vi "Day 14.vi"() -> ()   [LabVIEW 2025]
panel:
  out "# of sand":i32
  out "cave array":string[][](array[string])
  out "lines array":string[](array[string])
  out "sand pour":i32
  out "Y offset":i32
  out "X":i32
  out "Y":i32
  in  "test":bool
  in  "test input":string="498,4 -> 498,6 -> 496,6\n503,4 -> 502,4 -> 502,9 -> 494,9"
  in  "input":string="487,45 -> 487,38 -> 487,45 -> 489,45 -> 489,42 -> 489,45 -> 491,45 -> 491,39 -> 491,45 -> 493,45 -> 493,39 -> 493,45\n512,90 -> 512,87 -> 512,90 -> 514,90 -> 514,86 -> 514,90 -> 516,90 -> 516,87 -> 516,90 -> 518,90 -> 518,82 -> 518,90 -> 520,90 -> 520,81 -> 520,90 -> 522,90 -> 522,86 -> 522,90 -> 524,90 -> 524,84 -> 524,90 -> 526,90 -> 526,82 -> 526,90 -> 528,90 -> 528,82 -> 528,90\n494,16 -> 499,16\n512,90 -> 512,87 -> 512,90 -> 514,90 -> 514,86 -> 514,90 -> 516,90 -> 516,87 -> 516,90 -> 518,90 -> 518,82 -> 518,90 -> 520,90 -> 520,81 -> 520,90 -> 522,90 -> 522,86 -> 522,90 -> 524,90 -> 524,84 -> 524,90 -> 526,90 -> 526,82 -> 526,90 -> 528,90 -> 528,82 -> 528,90\n505,57 -> 505,59 -> 498,59 -> 498,66 -> 509,66 -> 509,59 -> 507,59 -> 507,57\n492,52 -> 496,52\n520,165 -> 520,160 -> 520,165 -> 522,165 -> 522,163 -> 522,165 -> 524,165 -> 524,159 -> 524,165 -> 526,165 -> 526,159 -> 526,165 -> 528,165 -> 528,155 -> 528,165\n510,123 -> 515,123\n492,48 -> 496,48\n512,90 -> 512,87 -> 512,90 -> 514,90 -> 514,86 -> 514,90 -> 516,90 -> 516,87 -> 516,90 -> 518,90 -> 518,82 -> 518,90 -> 520,90 -> 520,81 -> 520,90 -> 522,90 -> 522,86 -> 522,90 -> 524,90 -> 524,84 -> 524,90 -> 526,90 -> 526,82 -> 526,90 -> 528,90 -> 528,82 -> 528,90\n512,90 -> 512,87 -> 512,90 -> 514,90 -> 514,86 -> 514,90 -> 516,90 -> 516,87 -> 516,90 -> 518,90 -> 518,82 -> 518,90 -> 520,90 -> 520,81 -> 520,90 -> 522,90 -> 522,86 -> 522,90 -> 524,90 -> 524,84 -> 524,90 -> 526,90 -> 526,82 -> 526,90 -> 528,90 -> 528,82 -> 528,90\n487,45 -> 487,38 -> 487,45 -> 489,45 -> 489,42 -> 489,45 -> 491,45 -> 491,39 -> 491,45 -> 493,45 -> 493,39 -> 493,45\n501,54 -> 505,54\n513,120 -> 518,120\n502,138 -> 502,141 -> 498,141 -> 498,145 -> 514,145 -> 514,141 -> 507,141 -> 507,138\n483,54 -> 487,54\n505,57 -> 505,59 -> 498,59 -> 498,66 -> 509,66 -> 509,59 -> 507,59 -> 507,57\n508,103 -> 508,93 -> 508,103 -> 510,103 -> 510,101 -> 510,103 -> 512,103 -> 512,96 -> 512,103\n512,106 -> 512,108 -> 505,108 -> 505,114 -> 518,114 -> 518,108 -> 516,108 -> 516,106\n532,129 -> 537,129\n501,16 -> 506,16\n508,103 -> 508,93 -> 508,103 -> 510,103 -> 510,101 -> 510,103 -> 512,103 -> 512,96 -> 512,103\n502,138 -> 502,141 -> 498,141 -> 498,145 -> 514,145 -> 514,141 -> 507,141 -> 507,138\n520,120 -> 525,120\n489,50 -> 493,50\n498,19 -> 503,19\n505,151 -> 505,152 -> 518,152 -> 518,151\n510,73 -> 514,73\n516,77 -> 520,77\n487,45 -> 487,38 -> 487,45 -> 489,45 -> 489,42 -> 489,45 -> 491,45 -> 491,39 -> 491,45 -> 493,45 -> 493,39 -> 493,45\n520,165 -> 520,160 -> 520,165 -> 522,165 -> 522,163 -> 522,165 -> 524,165 -> 524,159 -> 524,165 -> 526,165 -> 526,159 -> 526,165 -> 528,165 -> 528,155 -> 528,165\n512,90 -> 512,87 -> 512,90 -> 514,90 -> 514,86 -> 514,90 -> 516,90 -> 516,87 -> 516,90 -> 518,90 -> 518,82 -> 518,90 -> 520,90 -> 520,81 -> 520,90 -> 522,90 -> 522,86 -> 522,90 -> 524,90 -> 524,84 -> 524,90 -> 526,90 -> 526,82 -> 526,90 -> 528,90 -> 528,82 -> 528,90\n511,129 -> 516,129\n512,90 -> 512,87 -> 512,90 -> 514,90 -> 514,86 -> 514,90 -> 516,90 -> 516,87 -> 516,90 -> 518,90 -> 518,82 -> 518,90 -> 520,90 -> 520,81 -> 520,90 -> 522,90 -> 522,86 -> 522,90 -> 524,90 -> 524,84 -> 524,90 -> 526,90 -> 526,82 -> 526,90 -> 528,90 -> 528,82 -> 528,90\n520,165 -> 520,160 -> 520,165 -> 522,165 -> 522,163 -> 522,165 -> 524,165 -> 524,159 -> 524,165 -> 526,165 -> 526,159 -> 526,165 -> 528,165 -> 528,155 -> 528,165\n512,90 -> 512,87 -> 512,90 -> 514,90 -> 514,86 -> 514,90 -> 516,90 -> 516,87 -> 516,90 -> 518,90 -> 518,82 -> 518,90 -> 520,90 -> 520,81 -> 520,90 -> 522,90 -> 522,86 -> 522,90 -> 524,90 -> 524,84 -> 524,90 -> 526,90 -> 526,82 -> 526,90 -> 528,90 -> 528,82 -> 528,90\n524,123 -> 529,123\n512,90 -> 512,87 -> 512,90 -> 514,90 -> 514,86 -> 514,90 -> 516,90 -> 516,87 -> 516,90 -> 518,90 -> 518,82 -> 518,90 -> 520,90 -> 520,81 -> 520,90 -> 522,90 -> 522,86 -> 522,90 -> 524,90 -> 524,84 -> 524,90 -> 526,90 -> 526,82 -> 526,90 -> 528,90 -> 528,82 -> 528,90\n505,57 -> 505,59 -> 498,59 -> 498,66 -> 509,66 -> 509,59 -> 507,59 -> 507,57\n487,45 -> 487,38 -> 487,45 -> 489,45 -> 489,42 -> 489,45 -> 491,45 -> 491,39 -> 491,45 -> 493,45 -> 493,39 -> 493,45\n520,165 -> 520,160 -> 520,165 -> 522,165 -> 522,163 -> 522,165 -> 524,165 -> 524,159 -> 524,165 -> 526,165 -> 526,159 -> 526,165 -> 528,165 -> 528,155 -> 528,165\n512,90 -> 512,87 -> 512,90 -> 514,90 -> 514,86 -> 514,90 -> 516,90 -> 516,87 -> 516,90 -> 518,90 -> 518,82 -> 518,90 -> 520,90 -> 520,81 -> 520,90 -> 522,90 -> 522,86 -> 522,90 -> 524,90 -> 524,84 -> 524,90 -> 526,90 -> 526,82 -> 526,90 -> 528,90 -> 528,82 -> 528,90\n507,75 -> 511,75\n495,22 -> 495,25 -> 492,25 -> 492,32 -> 501,32 -> 501,25 -> 499,25 -> 499,22\n514,149 -> 524,149 -> 524,148\n512,90 -> 512,87 -> 512,90 -> 514,90 -> 514,86 -> 514,90 -> 516,90 -> 516,87 -> 516,90 -> 518,90 -> 518,82 -> 518,90 -> 520,90 -> 520,81 -> 520,90 -> 522,90 -> 522,86 -> 522,90 -> 524,90 -> 524,84 -> 524,90 -> 526,90 -> 526,82 -> 526,90 -> 528,90 -> 528,82 -> 528,90\n504,129 -> 509,129\n487,45 -> 487,38 -> 487,45 -> 489,45 -> 489,42 -> 489,45 -> 491,45 -> 491,39 -> 491,45 -> 493,45 -> 493,39 -> 493,45\n520,165 -> 520,160 -> 520,165 -> 522,165 -> 522,163 -> 522,165 -> 524,165 -> 524,159 -> 524,165 -> 526,165 -> 526,159 -> 526,165 -> 528,165 -> 528,155 -> 528,165\n512,90 -> 512,87 -> 512,90 -> 514,90 -> 514,86 -> 514,90 -> 516,90 -> 516,87 -> 516,90 -> 518,90 -> 518,82 -> 518,90 -> 520,90 -> 520,81 -> 520,90 -> 522,90 -> 522,86 -> 522,90 -> 524,90 -> 524,84 -> 524,90 -> 526,90 -> 526,82 -> 526,90 -> 528,90 -> 528,82 -> 528,90\n508,103 -> 508,93 -> 508,103 -> 510,103 -> 510,101 -> 510,103 -> 512,103 -> 512,96 -> 512,103\n504,77 -> 508,77\n495,22 -> 495,25 -> 492,25 -> 492,32 -> 501,32 -> 501,25 -> 499,25 -> 499,22\n516,117 -> 521,117\n514,149 -> 524,149 -> 524,148\n512,90 -> 512,87 -> 512,90 -> 514,90 -> 514,86 -> 514,90 -> 516,90 -> 516,87 -> 516,90 -> 518,90 -> 518,82 -> 518,90 -> 520,90 -> 520,81 -> 520,90 -> 522,90 -> 522,86 -> 522,90 -> 524,90 -> 524,84 -> 524,90 -> 526,90 -> 526,82 -> 526,90 -> 528,90 -> 528,82 -> 528,90\n495,22 -> 495,25 -> 492,25 -> 492,32 -> 501,32 -> 501,25 -> 499,25 -> 499,22\n502,138 -> 502,141 -> 498,141 -> 498,145 -> 514,145 -> 514,141 -> 507,141 -> 507,138\n512,106 -> 512,108 -> 505,108 -> 505,114 -> 518,114 -> 518,108 -> 516,108 -> 516,106\n505,57 -> 505,59 -> 498,59 -> 498,66 -> 509,66 -> 509,59 -> 507,59 -> 507,57\n508,103 -> 508,93 -> 508,103 -> 510,103 -> 510,101 -> 510,103 -> 512,103 -> 512,96 -> 512,103\n508,103 -> 508,93 -> 508,103 -> 510,103 -> 510,101 -> 510,103 -> 512,103 -> 512,96 -> 512,103\n507,126 -> 512,126\n513,75 -> 517,75\n512,90 -> 512,87 -> 512,90 -> 514,90 -> 514,86 -> 514,90 -> 516,90 -> 516,87 -> 516,90 -> 518,90 -> 518,82 -> 518,90 -> 520,90 -> 520,81 -> 520,90 -> 522,90 -> 522,86 -> 522,90 -> 524,90 -> 524,84 -> 524,90 -> 526,90 -> 526,82 -> 526,90 -> 528,90 -> 528,82 -> 528,90\n502,138 -> 502,141 -> 498,141 -> 498,145 -> 514,145 -> 514,141 -> 507,141 -> 507,138\n505,151 -> 505,152 -> 518,152 -> 518,151\n510,77 -> 514,77\n528,126 -> 533,126\n520,165 -> 520,160 -> 520,165 -> 522,165 -> 522,163 -> 522,165 -> 524,165 -> 524,159 -> 524,165 -> 526,165 -> 526,159 -> 526,165 -> 528,165 -> 528,155 -> 528,165\n512,106 -> 512,108 -> 505,108 -> 505,114 -> 518,114 -> 518,108 -> 516,108 -> 516,106\n487,45 -> 487,38 -> 487,45 -> 489,45 -> 489,42 -> 489,45 -> 491,45 -> 491,39 -> 491,45 -> 493,45 -> 493,39 -> 493,45\n487,45 -> 487,38 -> 487,45 -> 489,45 -> 489,42 -> 489,45 -> 491,45 -> 491,39 -> 491,45 -> 493,45 -> 493,39 -> 493,45\n518,129 -> 523,129\n505,57 -> 505,59 -> 498,59 -> 498,66 -> 509,66 -> 509,59 -> 507,59 -> 507,57\n495,22 -> 495,25 -> 492,25 -> 492,32 -> 501,32 -> 501,25 -> 499,25 -> 499,22\n512,90 -> 512,87 -> 512,90 -> 514,90 -> 514,86 -> 514,90 -> 516,90 -> 516,87 -> 516,90 -> 518,90 -> 518,82 -> 518,90 -> 520,90 -> 520,81 -> 520,90 -> 522,90 -> 522,86 -> 522,90 -> 524,90 -> 524,84 -> 524,90 -> 526,90 -> 526,82 -> 526,90 -> 528,90 -> 528,82 -> 528,90\n512,90 -> 512,87 -> 512,90 -> 514,90 -> 514,86 -> 514,90 -> 516,90 -> 516,87 -> 516,90 -> 518,90 -> 518,82 -> 518,90 -> 520,90 -> 520,81 -> 520,90 -> 522,90 -> 522,86 -> 522,90 -> 524,90 -> 524,84 -> 524,90 -> 526,90 -> 526,82 -> 526,90 -> 528,90 -> 528,82 -> 528,90\n487,45 -> 487,38 -> 487,45 -> 489,45 -> 489,42 -> 489,45 -> 491,45 -> 491,39 -> 491,45 -> 493,45 -> 493,39 -> 493,45\n491,19 -> 496,19\n505,19 -> 510,19\n520,165 -> 520,160 -> 520,165 -> 522,165 -> 522,163 -> 522,165 -> 524,165 -> 524,159 -> 524,165 -> 526,165 -> 526,159 -> 526,165 -> 528,165 -> 528,155 -> 528,165\n508,103 -> 508,93 -> 508,103 -> 510,103 -> 510,101 -> 510,103 -> 512,103 -> 512,96 -> 512,103\n506,135 -> 517,135 -> 517,134\n487,45 -> 487,38 -> 487,45 -> 489,45 -> 489,42 -> 489,45 -> 491,45 -> 491,39 -> 491,45 -> 493,45 -> 493,39 -> 493,45\n506,135 -> 517,135 -> 517,134\n520,165 -> 520,160 -> 520,165 -> 522,165 -> 522,163 -> 522,165 -> 524,165 -> 524,159 -> 524,165 -> 526,165 -> 526,159 -> 526,165 -> 528,165 -> 528,155 -> 528,165\n487,45 -> 487,38 -> 487,45 -> 489,45 -> 489,42 -> 489,45 -> 491,45 -> 491,39 -> 491,45 -> 493,45 -> 493,39 -> 493,45\n512,106 -> 512,108 -> 505,108 -> 505,114 -> 518,114 -> 518,108 -> 516,108 -> 516,106\n512,90 -> 512,87 -> 512,90 -> 514,90 -> 514,86 -> 514,90 -> 516,90 -> 516,87 -> 516,90 -> 518,90 -> 518,82 -> 518,90 -> 520,90 -> 520,81 -> 520,90 -> 522,90 -> 522,86 -> 522,90 -> 524,90 -> 524,84 -> 524,90 -> 526,90 -> 526,82 -> 526,90 -> 528,90 -> 528,82 -> 528,90\n520,165 -> 520,160 -> 520,165 -> 522,165 -> 522,163 -> 522,165 -> 524,165 -> 524,159 -> 524,165 -> 526,165 -> 526,159 -> 526,165 -> 528,165 -> 528,155 -> 528,165\n497,13 -> 502,13\n489,54 -> 493,54\n512,90 -> 512,87 -> 512,90 -> 514,90 -> 514,86 -> 514,90 -> 516,90 -> 516,87 -> 516,90 -> 518,90 -> 518,82 -> 518,90 -> 520,90 -> 520,81 -> 520,90 -> 522,90 -> 522,86 -> 522,90 -> 524,90 -> 524,84 -> 524,90 -> 526,90 -> 526,82 -> 526,90 -> 528,90 -> 528,82 -> 528,90\n512,106 -> 512,108 -> 505,108 -> 505,114 -> 518,114 -> 518,108 -> 516,108 -> 516,106\n505,69 -> 505,70 -> 511,70 -> 511,69\n487,45 -> 487,38 -> 487,45 -> 489,45 -> 489,42 -> 489,45 -> 491,45 -> 491,39 -> 491,45 -> 493,45 -> 493,39 -> 493,45\n502,138 -> 502,141 -> 498,141 -> 498,145 -> 514,145 -> 514,141 -> 507,141 -> 507,138\n520,165 -> 520,160 -> 520,165 -> 522,165 -> 522,163 -> 522,165 -> 524,165 -> 524,159 -> 524,165 -> 526,165 -> 526,159 -> 526,165 -> 528,165 -> 528,155 -> 528,165\n512,106 -> 512,108 -> 505,108 -> 505,114 -> 518,114 -> 518,108 -> 516,108 -> 516,106\n512,90 -> 512,87 -> 512,90 -> 514,90 -> 514,86 -> 514,90 -> 516,90 -> 516,87 -> 516,90 -> 518,90 -> 518,82 -> 518,90 -> 520,90 -> 520,81 -> 520,90 -> 522,90 -> 522,86 -> 522,90 -> 524,90 -> 524,84 -> 524,90 -> 526,90 -> 526,82 -> 526,90 -> 528,90 -> 528,82 -> 528,90\n520,165 -> 520,160 -> 520,165 -> 522,165 -> 522,163 -> 522,165 -> 524,165 -> 524,159 -> 524,165 -> 526,165 -> 526,159 -> 526,165 -> 528,165 -> 528,155 -> 528,165\n525,129 -> 530,129\n512,90 -> 512,87 -> 512,90 -> 514,90 -> 514,86 -> 514,90 -> 516,90 -> 516,87 -> 516,90 -> 518,90 -> 518,82 -> 518,90 -> 520,90 -> 520,81 -> 520,90 -> 522,90 -> 522,86 -> 522,90 -> 524,90 -> 524,84 -> 524,90 -> 526,90 -> 526,82 -> 526,90 -> 528,90 -> 528,82 -> 528,90\n512,90 -> 512,87 -> 512,90 -> 514,90 -> 514,86 -> 514,90 -> 516,90 -> 516,87 -> 516,90 -> 518,90 -> 518,82 -> 518,90 -> 520,90 -> 520,81 -> 520,90 -> 522,90 -> 522,86 -> 522,90 -> 524,90 -> 524,84 -> 524,90 -> 526,90 -> 526,82 -> 526,90 -> 528,90 -> 528,82 -> 528,90\n505,151 -> 505,152 -> 518,152 -> 518,151\n495,22 -> 495,25 -> 492,25 -> 492,32 -> 501,32 -> 501,25 -> 499,25 -> 499,22\n521,126 -> 526,126\n512,106 -> 512,108 -> 505,108 -> 505,114 -> 518,114 -> 518,108 -> 516,108 -> 516,106\n495,50 -> 499,50\n495,54 -> 499,54\n502,138 -> 502,141 -> 498,141 -> 498,145 -> 514,145 -> 514,141 -> 507,141 -> 507,138\n512,90 -> 512,87 -> 512,90 -> 514,90 -> 514,86 -> 514,90 -> 516,90 -> 516,87 -> 516,90 -> 518,90 -> 518,82 -> 518,90 -> 520,90 -> 520,81 -> 520,90 -> 522,90 -> 522,86 -> 522,90 -> 524,90 -> 524,84 -> 524,90 -> 526,90 -> 526,82 -> 526,90 -> 528,90 -> 528,82 -> 528,90\n508,103 -> 508,93 -> 508,103 -> 510,103 -> 510,101 -> 510,103 -> 512,103 -> 512,96 -> 512,103\n512,90 -> 512,87 -> 512,90 -> 514,90 -> 514,86 -> 514,90 -> 516,90 -> 516,87 -> 516,90 -> 518,90 -> 518,82 -> 518,90 -> 520,90 -> 520,81 -> 520,90 -> 522,90 -> 522,86 -> 522,90 -> 524,90 -> 524,84 -> 524,90 -> 526,90 -> 526,82 -> 526,90 -> 528,90 -> 528,82 -> 528,90\n508,103 -> 508,93 -> 508,103 -> 510,103 -> 510,101 -> 510,103 -> 512,103 -> 512,96 -> 512,103\n512,90 -> 512,87 -> 512,90 -> 514,90 -> 514,86 -> 514,90 -> 516,90 -> 516,87 -> 516,90 -> 518,90 -> 518,82 -> 518,90 -> 520,90 -> 520,81 -> 520,90 -> 522,90 -> 522,86 -> 522,90 -> 524,90 -> 524,84 -> 524,90 -> 526,90 -> 526,82 -> 526,90 -> 528,90 -> 528,82 -> 528,90\n495,22 -> 495,25 -> 492,25 -> 492,32 -> 501,32 -> 501,25 -> 499,25 -> 499,22\n498,52 -> 502,52\n517,123 -> 522,123\n514,126 -> 519,126\n512,90 -> 512,87 -> 512,90 -> 514,90 -> 514,86 -> 514,90 -> 516,90 -> 516,87 -> 516,90 -> 518,90 -> 518,82 -> 518,90 -> 520,90 -> 520,81 -> 520,90 -> 522,90 -> 522,86 -> 522,90 -> 524,90 -> 524,84 -> 524,90 -> 526,90 -> 526,82 -> 526,90 -> 528,90 -> 528,82 -> 528,90\n512,90 -> 512,87 -> 512,90 -> 514,90 -> 514,86 -> 514,90 -> 516,90 -> 516,87 -> 516,90 -> 518,90 -> 518,82 -> 518,90 -> 520,90 -> 520,81 -> 520,90 -> 522,90 -> 522,86 -> 522,90 -> 524,90 -> 524,84 -> 524,90 -> 526,90 -> 526,82 -> 526,90 -> 528,90 -> 528,82 -> 528,90\n495,22 -> 495,25 -> 492,25 -> 492,32 -> 501,32 -> 501,25 -> 499,25 -> 499,22\n505,69 -> 505,70 -> 511,70 -> 511,69\n520,165 -> 520,160 -> 520,165 -> 522,165 -> 522,163 -> 522,165 -> 524,165 -> 524,159 -> 524,165 -> 526,165 -> 526,159 -> 526,165 -> 528,165 -> 528,155 -> 528,165\n512,90 -> 512,87 -> 512,90 -> 514,90 -> 514,86 -> 514,90 -> 516,90 -> 516,87 -> 516,90 -> 518,90 -> 518,82 -> 518,90 -> 520,90 -> 520,81 -> 520,90 -> 522,90 -> 522,86 -> 522,90 -> 524,90 -> 524,84 -> 524,90 -> 526,90 -> 526,82 -> 526,90 -> 528,90 -> 528,82 -> 528,90\n520,165 -> 520,160 -> 520,165 -> 522,165 -> 522,163 -> 522,165 -> 524,165 -> 524,159 -> 524,165 -> 526,165 -> 526,159 -> 526,165 -> 528,165 -> 528,155 -> 528,165\n505,57 -> 505,59 -> 498,59 -> 498,66 -> 509,66 -> 509,59 -> 507,59 -> 507,57\n520,165 -> 520,160 -> 520,165 -> 522,165 -> 522,163 -> 522,165 -> 524,165 -> 524,159 -> 524,165 -> 526,165 -> 526,159 -> 526,165 -> 528,165 -> 528,155 -> 528,165\n505,69 -> 505,70 -> 511,70 -> 511,69\n505,57 -> 505,59 -> 498,59 -> 498,66 -> 509,66 -> 509,59 -> 507,59 -> 507,57\n502,138 -> 502,141 -> 498,141 -> 498,145 -> 514,145 -> 514,141 -> 507,141 -> 507,138\n486,52 -> 490,52\n"
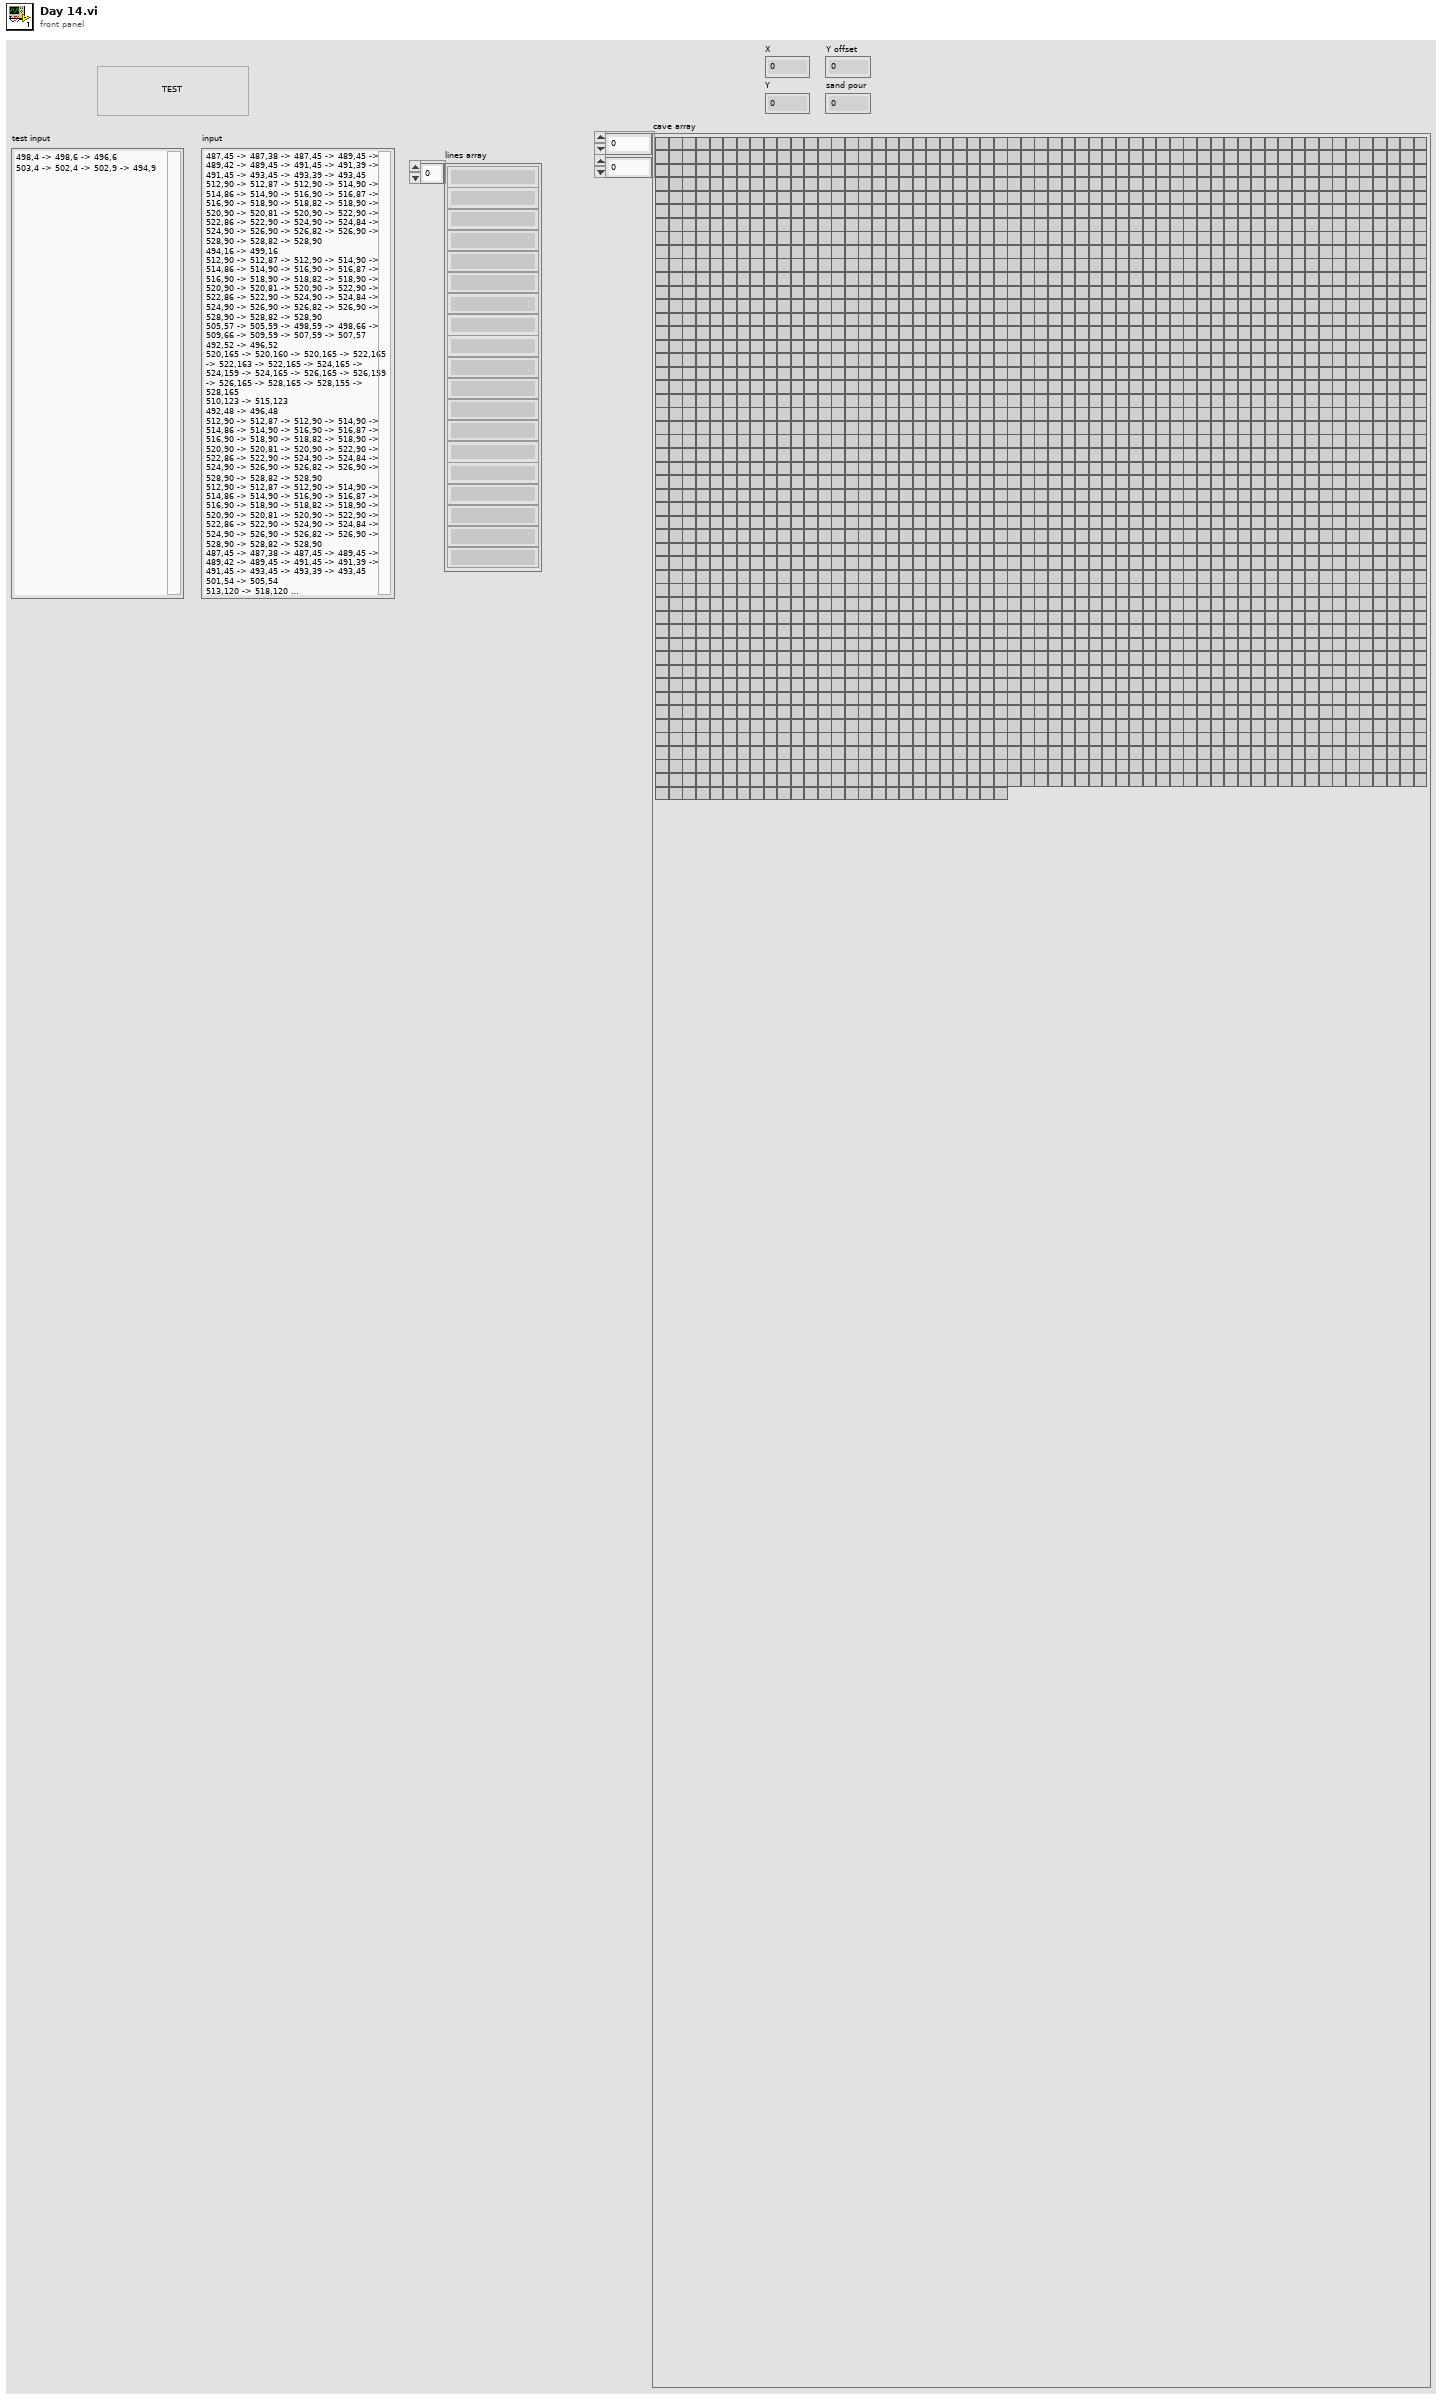
[diagram p1: front panel]
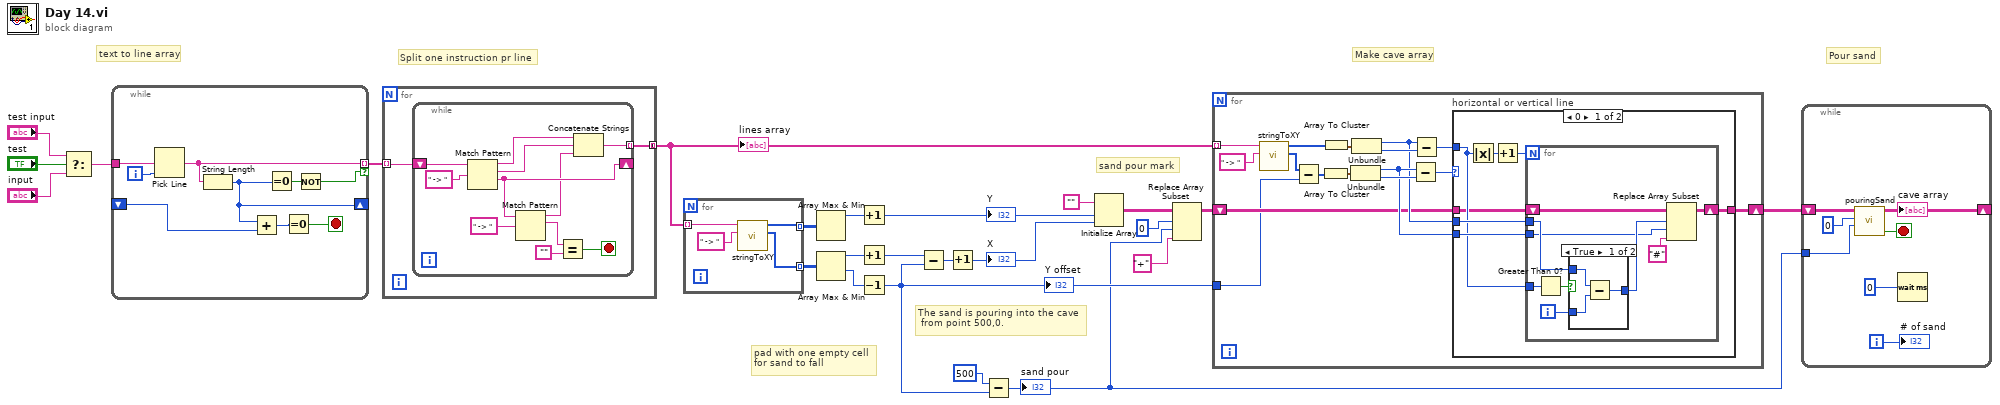
[diagram p0: block diagram]
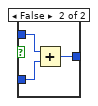
[diagram p2: hidden frame]
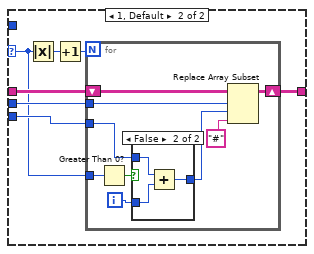
[diagram p3: hidden frame]
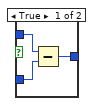
[diagram p4: hidden frame]
diagram:
  # "The sand is pouring into the cave\n from point 500,0."
  # "Pour sand"
  # "Split one instruction pr line"
  # "pad with one empty cell\nfor sand to fall"
  # "Make cave array"
  # "sand pour mark"
  # "text to line array"
  n1 = Select(t="test input", s="test", f="input") -> (s? t:f=w21:string)
  n2 = while {
    tunnel: w21 -> [w32]
    tunnel: [w25] -> w18 mode=indexing if=w31
    shift-right: [w28] -> _
    shift-left: _ -> [w29]
    i -> [w33]
    stop <- w26 stop-if-true
    n3 = Pick Line(multi-line string=w32, line index=w33) -> (output string=w25:string)  [unwired: 1 in]
    n4 = String Length(string=w25) -> (length=w28:i32)
    n5 = Add(x=w28, y=w29) -> (x+y=w30:i32)
    n6 = Equal To 0?(x=w28) -> (x = 0?=w27:bool)
    n7 = Equal To 0?(x=w30) -> (x = 0?=w26:bool)
    n8 = Not(x=w27) -> (.not. x?=w31:bool)
  }
  n9 = for {
    tunnel: w18 -> [w35] mode=indexing
    tunnel: [w34] -> w6 mode=concatenating
    n10 = while {
      shift-right: [w43] -> _
      shift-left: w35 -> [w45]
      tunnel: [w40] -> w34 mode=indexing
      stop <- w37 stop-if-true
      n11 = Match Pattern(string=w45, regular expression=" -> " ("delimiter")) -> (before substring=w42:string, match substring=w41:string, after substring=w43:string)  [unwired: 1 in, 1 out]
      n12 = Match Pattern(string=w43, regular expression=" -> " ("delimiter")) -> (before substring=w36:string, match substring=w38:string)  [unwired: 1 in, 2 out]
      n13 = Equal?(x=w38, y="") -> (x = y?=w37:bool)
      n14 = Concatenate Strings(w42, w41, w36) -> (w40:string)
    }
  }
  "lines array" <- w6
  n15 = for {
    tunnel: w6 -> [w49] mode=indexing
    tunnel: [w48] -> w5 mode=indexing
    tunnel: [w47] -> w4 mode=indexing
    n16 = call "stringToXY.vi"("delimiter"=" -> ", "string"=w49) -> ("X"=w47:i32[], "Y"=w48:i32[])  [unwired: 8 in]
  }
  n17 = Array Max & Min(array=w5) -> (max value=w3:i32)  [unwired: 3 out]
  n18 = Array Max & Min(array=w4) -> (max value=w2:i32, min value=w1:i32)  [unwired: 2 out]
  n19 = Increment(x=w3) -> (x+1=w7:i32)
  "Y" <- w7
  n20 = Increment(x=w2) -> (x+1=w13:i32)
  n21 = Decrement(x=w1) -> (x-1=w12:i32)
  "Y offset" <- w12
  n22 = Subtract(x=w13, y=w12) -> (x-y=w17:i32)
  n23 = Increment(x=w17) -> (x+1=w15:i32)
  "X" <- w15
  n24 = Subtract(x=500, y=w12) -> (x-y=w9:i32)
  "sand pour" <- w9
  n25 = Initialize Array("", w7, w15) -> (w11:string[][])
  n26 = Replace Array Subset(array=w11, new element="+" ("new element/subarray"), index (row)=0 ("index (col)"), index (col)=w9) -> (w8:string[][])
  n27 = for {
    tunnel: w6 -> [w54] mode=indexing
    shift-right: [w57] -> w10
    shift-left: w8 -> [w56]
    tunnel: w12 -> [w53]
    n28 = call "stringToXY.vi"("delimiter"=" -> ", "string"=w54) -> ("X"=w52:i32[], "Y"=w51:i32[])  [unwired: 8 in]
    n29 = Subtract(x=w52, y=w53) -> (x-y=w55:i32[])
    n30 = Array To Cluster(array=w55) -> (cluster=w65:cluster{"[0]":i32, "[1]":i32})
    n31 = Array To Cluster(array=w51) -> (cluster=w64:cluster{"Y[0]":i32, "Y[1]":i32})
    n32 = Unbundle(w65) -> ("[0]"=w59:i32, "[1]"=w63:i32)
    n33 = Unbundle(w64) -> ("Y[0]"=w58:i32, "Y[1]"=w61:i32)
    n34 = Subtract(x=w59, y=w63) -> (x-y=w62:i32)
    n35 = Subtract(x=w58, y=w61) -> (x-y=w60:i32)
    n36 = case "horizontal or vertical line" shown="0" w62 {
      selector: w62 -> [_ w90]
      tunnel: w60 -> [w70 _]
      tunnel: w59 -> [w72 w94]
      tunnel: w58 -> [w71 w93]
      tunnel: [w69 w92] -> w57
      tunnel: w56 -> [w68 w91]
      frame 0 {
        n37 = Absolute Value(x=w70) -> (abs(x)=w73:i32)
        n38 = Increment(x=w73) -> (x+1=w67:i32)
        n39 = for {
          N: w67 -> [_]
          tunnel: w72 -> [w74]
          tunnel: w71 -> [w81]
          tunnel: w70 -> [w82]
          shift-right: [w78] -> w69
          shift-left: w68 -> [w79]
          i -> [w80]
          n40 = Greater Than 0?(x=w82) -> (x > 0?=w77:bool)
          n41 = case shown="True" w77 {
            tunnel: w81 -> [w85 w88]
            tunnel: w80 -> [w84 w87]
            tunnel: [w83 w86] -> w76
            frame True {
              n42 = Subtract(x=w85, y=w84) -> (x-y=w83:i32)
            }
            frame False {
              n43 = Add(x=w88, y=w87) -> (x+y=w86:i32)
            }
          }
          n44 = Replace Array Subset(array=w79, new element="#" ("new element/subarray"), index (row)=w76, index (col)=w74) -> (w78:string[][])
        }
      }
      frame 1, Default {
        n45 = Absolute Value(x=w90) -> (abs(x)=w95:i32)
        n46 = Increment(x=w95) -> (x+1=w89:i32)
        n47 = for {
          N: w89 -> [_]
          tunnel: w94 -> [w99]
          tunnel: w93 -> [w97]
          tunnel: w90 -> [w103]
          shift-right: [w100] -> w92
          shift-left: w91 -> [w101]
          i -> [w102]
          n48 = Greater Than 0?(x=w103) -> (x > 0?=w104:bool)
          n49 = case shown="False" w104 {
            tunnel: w99 -> [w107 w110]
            tunnel: w102 -> [w106 w109]
            tunnel: [w105 w108] -> w96
            frame True {
              n50 = Subtract(x=w107, y=w106) -> (x-y=w105:i32)
            }
            frame False {
              n51 = Add(x=w110, y=w109) -> (x+y=w108:i32)
            }
          }
          n52 = Replace Array Subset(array=w101, new element="#" ("new element/subarray"), index (row)=w97, index (col)=w96) -> (w100:string[][])
        }
      }
    }
  }
  n53 = while {
    tunnel: w9 -> [w113]
    shift-right: [w112] -> _
    shift-left: w10 -> [w115]
    i -> [w111]
    stop <- w117 stop-if-true
    n54 = call "pouringSand.vi"("sand pour"=w113, "Y"=0, "cave"=w115) -> ("escape"=w117:bool, "cave"=w112:string[][])  [unwired: 7 in]
    "cave array" <- w112
    n55 = Wait (ms)(milliseconds to wait=u32 0 ("50")) -> ()  [unwired: 1 out]
    "# of sand" <- w111
  }
